vi "niScope Setup Virtual Channels.vi"(4 "samples count":i64=50000 min=1, 6 "fs [Hz]":dbl=50000.0, 7 "trigger setup (Immediate)":T1={"coupling"=1, "level [V]"=0.0, "slope"=0, "mode"=enum."Immediate"} {"level [V]" format="%.2f"; "coupling" items=["AC"=0, "DC"=1, "HF Reject"=3, "LF Reject"=4, "AC Plus HF Reject"=1001]}, 8 "error in":errorcluster, 10 "voltage ranges [Vpk] (empty: use global default)":dbl[](array[numeric]), 11 "niScope in":T4={"channel cfg"=[], "sessions"=[], "multi cards"=FALSE, "channels"=0, "type"=enum."n/a", "memory [B/chn]"=0, "ext. clock [Hz]"=0.0, "samples count"=0, "use streaming"=FALSE, "proc setup"={"packet size [smpl]"=0, "current timeout [s]"=0.0, "blk2blk timeout [s]"=0.0, "event time"=timestamp(0 s since 1904-01-01), "temp sampl T [s]"=0.0, "data queue"=refnum, "stop notifier"=refnum, "proc ref"=refnum}, "sample width [B]"=0, "ranges [V]"=[], "trigger setup"={"coupling"=1, "level [V]"=0.0, "slope"=0, "mode"=enum."Immediate"}, "fs [Hz]"=0.0, "bitres [bit]"=0} {"trigger setup"."level [V]" format="%.2f"; "trigger setup"."coupling" items=["AC"=0, "DC"=1, "HF Reject"=3, "LF Reject"=4, "AC Plus HF Reject"=1001]; "channel cfg"."Range [Vpk]" min=0.0; "channel cfg"."Channel" min=0}) -> (0 "error out":errorcluster, 3 "niScope out":T4={"channel cfg"=[], "sessions"=[], "multi cards"=FALSE, "channels"=0, "type"=enum."n/a", "memory [B/chn]"=0, "ext. clock [Hz]"=0.0, "samples count"=0, "use streaming"=FALSE, "proc setup"={"packet size [smpl]"=0, "current timeout [s]"=0.0, "blk2blk timeout [s]"=0.0, "event time"=timestamp(0 s since 1904-01-01), "temp sampl T [s]"=0.0, "data queue"=refnum, "stop notifier"=refnum, "proc ref"=refnum}, "sample width [B]"=0, "ranges [V]"=[], "trigger setup"={"coupling"=1, "level [V]"=0.0, "slope"=0, "mode"=enum."Immediate"}, "fs [Hz]"=0.0, "bitres [bit]"=0} {"trigger setup"."level [V]" format="%.2f"; "trigger setup"."coupling" items=["AC"=0, "DC"=1, "HF Reject"=3, "LF Reject"=4, "AC Plus HF Reject"=1001]; "channel cfg"."Range [Vpk]" min=0.0; "channel cfg"."Channel" min=0})   [LabVIEW 2018, in "niScope Virtual Digitizer.lvlib"]
doc: "Configures all virtual channels of the digitizer. Uses global and channel settings from the input session. If vector of voltage ranges in assigned to the function it will override default channel setting from the session. If it is empty, the defaults in the session will be used. Sampling rate and samples count to capture are set by additional inputs. Trigger can be set to other than immediate mode only for single shot mode (for streaming mode it is not yet supported). The VI prepares the cards for acquiring the data. It also implements synchronization via ni-Tclk in case multiple cards are used together. Call this at least once before doing first acquisition. It is not necessary to call this again when multiple acquisitions are performed repetedely with identical settings."
uses:
  niScope Virtual Digitizer.lvlib
  niScope Session.ctl
  niScope Virtual Channel Config.ctl
  niScope Virtual Channel Mode.ctl
  niScope Virtual Channel Input Z.ctl
  niScope Virtual Channel Coupling.ctl
  niScope Type.ctl
  niScope Digitizing Process Options.ctl
  niScope Data Packet.ctl
  niScope Trigger Setup.ctl
  <instrlib>/niScope/Controls/niScope trigger coupling.ctl
  <instrlib>/niScope/Controls/niScope trigger slope.ctl
  <instrlib>/niScope/Controls/niScope vertical coupling.ctl
  <instrlib>/niScope/Controls/niScope trigger source.ctl
  <vilib>/Utility/error.llb/Error Cluster From Error Code.vi
  <instrlib>/niScope/Configure/Trigger/niScope Configure Trigger Edge.vi
  <instrlib>/niScope/Configure/Trigger/niScope Configure Trigger Immediate.vi
  <instrlib>/niScope/Configure/Trigger/niScope Configure Trigger Software.vi
  <vilib>/ErrorRing/Error Ring.xnode
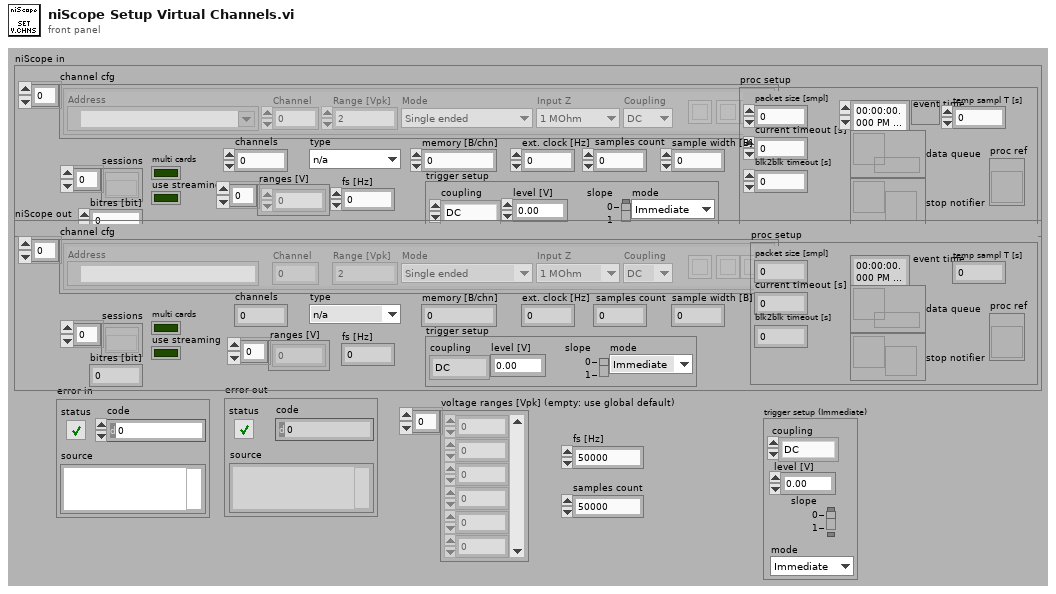
[diagram p1: front panel]
types:
  T1 = typedef "niScope Virtual Digitizer.lvlib/niScope Trigger Setup.ctl" = cluster{"coupling":T2, "level [V]":dbl, "slope":T3, "mode":enum16{"Immediate", "External", "Level"}}
  T2 = typedef "niScope trigger coupling.ctl" = u16
  T3 = typedef "niScope trigger slope.ctl" = i32
  T4 = typedef "niScope Virtual Digitizer.lvlib/niScope Session.ctl" = cluster{"channel cfg":T5[], "sessions":refnum<k20>[], "multi cards":bool, "channels":i32, "type":T9, "memory [B/chn]":i32, "ext. clock [Hz]":dbl, "samples count":i64, "use streaming":bool, "proc setup":T10, "sample width [B]":i32, "ranges [V]":dbl[], "trigger setup":T1, "fs [Hz]":dbl, "bitres [bit]":i32}
  T5 = typedef "niScope Virtual Digitizer.lvlib/niScope Virtual Channel Config.ctl" = cluster{"Address":refnum<k15>, "Channel":i32, "Mode":T6, "Input Z":T7, "Coupling":T8, "Range [Vpk]":dbl, "btn clr":bool, "btn up":bool, "btn down":bool}
  T6 = typedef "niScope Virtual Digitizer.lvlib/niScope Virtual Channel Mode.ctl" = enum16{"Single ended", "Unbal. differential", "Differential"}
  T7 = typedef "niScope Virtual Digitizer.lvlib/niScope Virtual Channel Input Z.ctl" = enum16{"1 MOhm", "50 Ohm"}
  T8 = typedef "niScope Virtual Digitizer.lvlib/niScope Virtual Channel Coupling.ctl" = enum16{"AC", "DC", "GND"}
  T9 = typedef "niScope Virtual Digitizer.lvlib/niScope Type.ctl" = enum16{"n/a", "5922"}
  T10 = typedef "niScope Virtual Digitizer.lvlib/niScope Digitizing Process Options.ctl" = cluster{"packet size [smpl]":i64, "current timeout [s]":dbl, "blk2blk timeout [s]":dbl, "event time":timestamp, "temp sampl T [s]":dbl, "data queue":refnum<queue>, "stop notifier":refnum<notifier>, "proc ref":refnum<vi>}
  T11 = typedef "niScope Virtual Digitizer.lvlib/niScope Physical Cards.ctl" = cluster{"chn lst":i32[], "addr":refnum<k15>, "chn pos":i32[]}
  T12 = typedef "niScope trigger source.ctl" = string
  T13 = typedef "niScope vertical coupling.ctl" = i32
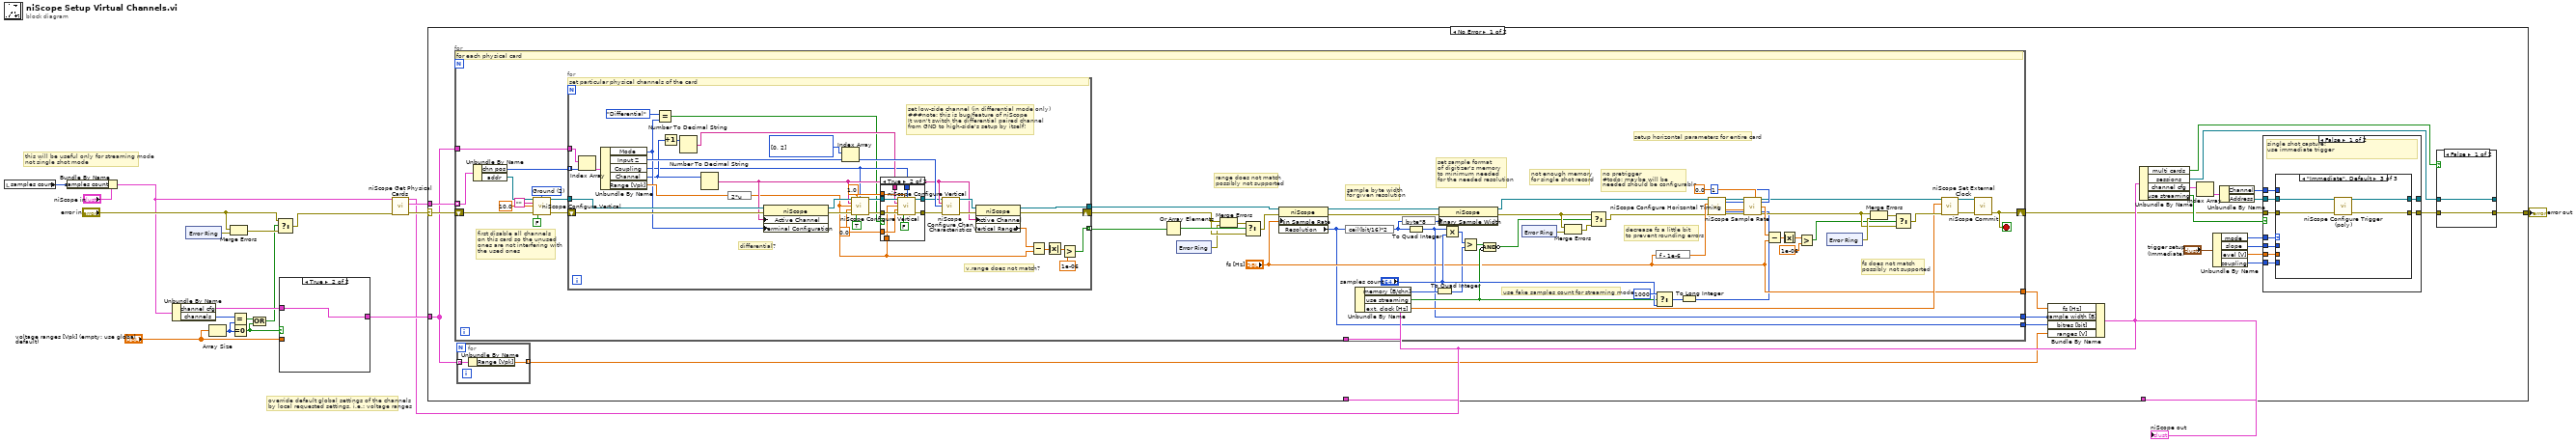
[diagram p0: block diagram]
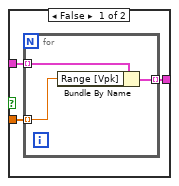
[diagram p2: hidden frame]
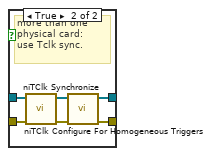
[diagram p3: hidden frame]
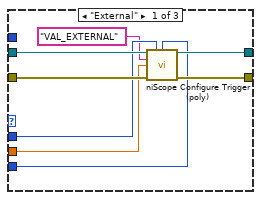
[diagram p4: hidden frame]
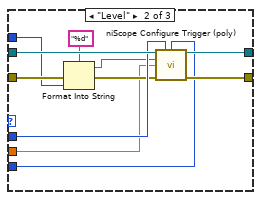
[diagram p5: hidden frame]
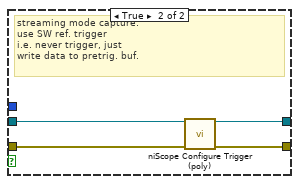
[diagram p6: hidden frame]
diagram:
  # "this will be useful only for streaming mode\nnot single shot mode"
  # "override default global settings of the channels\nby local requested settings, i.e.: voltage ranges"
  n1 = local read "samples count"() -> (w11:i64)
  n2 = Bundle By Name(cluster="niScope in", "samples count"=w11) -> (w9:T4)
  n3 = Unbundle By Name(w9) -> ("channel cfg"=w18:T5[], "channels"=w19:i32)
  n4 = xnode "Error Ring"() -> ("error out"=w15:errorcluster)
  n5 = Array Size(array="voltage ranges [Vpk] (empty: use global default)") -> (size(s)=w6:i32)
  n6 = Merge Errors("error in", w15) -> (w14:errorcluster)
  n7 = Equal?(x=w19, y=w6) -> (x = y?=w7:bool)
  n8 = Equal To 0?(x=w6) -> (x = 0?=w3:bool)
  n9 = Compound Arithmetic op=OR(w7, w3) -> (w5:bool)
  n10 = Select(t="error in", s=w5, f=w14) -> (s? t:f=w2:errorcluster)
  n11 = case shown="True" w3 {
    tunnel: w18 -> [w23 w27]
    tunnel: [w22 w27] -> w17
    tunnel: "voltage ranges [Vpk] (empty: use global default)" -> [w21 _]
    frame False {
      n12 = for {
        tunnel: w23 -> [w26] mode=indexing
        tunnel: w21 -> [w24] mode=indexing
        tunnel: [w25] -> w22 mode=indexing
        n13 = Bundle By Name(cluster=w26, "Range [Vpk]"=w24) -> (w25:T5)
      }
    }
    frame True {
    }
  }
  n14 = call "niScope Get Physical Cards.vi"("error in"=w2, "niScope in"=w9) -> ("error out"=w13:errorcluster, "card list"=w20:T11[], "niScope out"=w8:T4)  [unwired: 7 in]
  n15 = case shown="No Error" w13 {
    selector: w13 -> [w51 w222]
    tunnel: w20 -> [w33 _]
    tunnel: w17 -> [w32 _]
    tunnel: w8 -> [w36 w221]
    tunnel: [w43 w222] -> w10
    tunnel: [w35 w221] -> w1
    frame No Error {
      n16 = for {
        tunnel: w33 -> [w157] mode=indexing
        shift-right: [w128] -> w28
        shift-left: w51 -> [w154]
        tunnel: w32 -> [w148]
        tunnel: w36 -> [w138]
        tunnel: [w102] -> w34
        tunnel: ["fs [Hz]"] -> w30
        tunnel: [w99] -> w29
        stop <- w128 stop-if-true
        w150 = T13 2 items=["AC", "DC", "Ground"] ("vertical coupling")
        # "set sample format\nof digitizer's memory\nto minimum needed\nfor the needed resolution"
        # "not enough memory\nfor single shot record"
        # "sample byte width\nfor given resolution"
        # "use fake samples count for streaming mode"
        # "fs does not match\npossibly not supported"
        # "setup horizontal parameters for entire card"
        # "range does not match\npossibly not supported"
        # "decrease fs a little bit\nto prevent rounding errors"
        # "no pretrigger\n#todo: maybe will be\nneeded should be configurable"
        # "first disable all channels\non this card so the unused\nones are not interfering with\nthe used ones"
        # "for each physical card"
        n17 = Unbundle By Name(w157) -> ("chn pos"=w156:i32[], "addr"=w153:refnum<k15>)
        n18 = call <instrlib>:"niScope Configure Vertical.vi"("instrument handle"=w153, "vertical coupling"=w150, "channels"="", "vertical range"=10.0, "error in"=w154, "channel enabled"=FALSE) -> ("instrument handle out"=w152:refnum<k15>, "error out"=w155:errorcluster)  [unwired: 8 in]
        n19 = for {
          shift-right: [w193] -> w134
          shift-left: w155 -> [w202]
          tunnel: w156 -> [w208] mode=indexing
          tunnel: w152 -> [w201]
          tunnel: w148 -> [w204]
          tunnel: [w192] -> w119
          tunnel: [w191] -> w137 mode=indexing
          w189 = u32[] [0, 2] items=["1 mega ohm"=0, "50 ohms"=2]
          w175 = 0.0 ("vertical offset")
          w177 = 1.0 ("probe attenuation")
          # "set low-side channel (in differential mode only)\n###note: this is bug/feature of niScope\nIt won't switch the differential paired channel\nfrom GND to high-side's setup by itself!"
          # "v.range does not match?"
          # "differential?"
          # "set particular physical channels of the card"
          n20 = Index Array(array=w204, index=w208) -> (element=w207:T5)
          n21 = Unbundle By Name(w207) -> ("Mode"=w187:T6, "Input Z"=w190:T7, "Coupling"=w176:T8, "Channel"=w185:i32, "Range [Vpk]"=w206:dbl)
          n22 = Equal?(x=niScope_Virtual_Channel_Mode."Differential", y=w187) -> (x = y?=w173:bool)
          n23 = Increment(x=w185) -> (x+1=w183:i32)
          n24 = Number To Decimal String(number=w183) -> (decimal integer string=w178:string)  [unwired: 1 in]
          n25 = Number To Decimal String(number=w185) -> (decimal integer string=w184:string)  [unwired: 1 in]
          n26 = expression code="2*u"(w206) -> (w174:dbl)
          n27 = property class="niScope"(reference=w201, error in=w202, "Active Channel"=w184, "Terminal Configuration"=w187) -> (reference out=w200:refnum<k15>, error out=w203:errorcluster)
          n28 = Index Array(array=w189, index=w190) -> (element=w188:u32)
          n29 = call <instrlib>:"niScope Configure Vertical.vi"("instrument handle"=w200, "probe attenuation"=w177, "vertical coupling"=w176, "channels"=w184, "vertical range"=w174, "vertical offset"=w175, "error in"=w203, "channel enabled"=TRUE) -> ("instrument handle out"=w181:refnum<k15>, "error out"=w182:errorcluster)  [unwired: 6 in]
          n30 = case shown="True" w173 {
            tunnel: w182 -> [w209 w220]
            tunnel: w181 -> [w210 w219]
            tunnel: [w209 w218] -> w180
            tunnel: [w210 w217] -> w179
            tunnel: w178 -> [_ w216]
            tunnel: w177 -> [_ w215]
            tunnel: w176 -> [_ w214]
            tunnel: w175 -> [_ w212]
            tunnel: w174 -> [_ w211]
            frame False {
            }
            frame True {
              n31 = call <instrlib>:"niScope Configure Vertical.vi"("instrument handle"=w219, "probe attenuation"=w215, "vertical coupling"=w214, "channels"=w216, "vertical range"=w211, "vertical offset"=w212, "error in"=w220, "channel enabled"=FALSE) -> ("instrument handle out"=w217:refnum<k15>, "error out"=w218:errorcluster)  [unwired: 6 in]
            }
          }
          n32 = call <instrlib>:"niScope Configure Chan Characteristics.vi"("instrument handle"=w179, "channels"=w184, "input impedance"=w188, "error in"=w180) -> ("instrument handle out"=w198:refnum<k15>, "error out"=w199:errorcluster)  [unwired: 10 in]
          n33 = property class="niScope"(reference=w198, error in=w199, "Active Channel"=w184) -> (reference out=w192:refnum<k15>, error out=w193:errorcluster, "Vertical Range"=w197:dbl)
          n34 = Subtract(x=w197, y=w174) -> (x-y=w196:dbl)
          n35 = Absolute Value(x=w196) -> (abs(x)=w195:dbl)
          n36 = Greater?(x=w195, y=1e-06) -> (0:w191:bool)
        }
        n37 = Or Array Elements(Boolean array=w137) -> (logical OR=w136:bool)
        n38 = xnode "Error Ring"() -> ("error out"=w133:errorcluster)
        n39 = Merge Errors(w134, w133) -> (w135:errorcluster)
        n40 = Select(t=w135, s=w136, f=w134) -> (s? t:f=w120:errorcluster)
        n41 = property class="niScope"(reference=w119, error in=w120, "Min Sample Rate"="fs [Hz]") -> (reference out=w109:refnum<k15>, error out=w110:errorcluster, "Resolution"=w99:i32)
        n42 = expression code="ceil(bit/16)*2"(w99) -> (w104:i32)
        n43 = Unbundle By Name(w138) -> ("memory [B/chn]"=w114:i32, "use streaming"=w112:bool, "ext. clock [Hz]"=w124:dbl)
        n44 = expression code="byte*8"(w104) -> (w108:i32)
        n45 = To Quad Integer(1:w104) -> (0:w102:i64)
        n46 = To Quad Integer(1:w114) -> (0:w101:i64)
        n47 = property class="niScope"(reference=w109, error in=w110, "Binary Sample Width"=w108) -> (reference out=w106:refnum<k15>, error out=w107:errorcluster)
        n48 = Multiply(x=w102, y="samples count") -> (x*y=w115:i64)
        n49 = Greater?(x=w115, y=w101) -> (0:w113:bool)
        n50 = Compound Arithmetic op=AND(w113, invert w112) -> (invert w105:bool)
        n51 = xnode "Error Ring"() -> ("error out"=w117:errorcluster)
        n52 = Merge Errors(w107, w117) -> (w118:errorcluster)
        n53 = Select(t=w107, s=w105, f=w118) -> (s? t:f=w111:errorcluster)
        n54 = expression code="f - 1e-6"("fs [Hz]") -> (w143:dbl)
        n55 = Select(t=i64 1000, s=w112, f="samples count") -> (s? t:f=w122:i64)
        n56 = To Long Integer(number=w122) -> (32bit integer=w100:i32)
        n57 = call <instrlib>:"niScope Configure Horizontal Timing.vi"("instrument handle"=w106, "number of records"=1, "min sample rate"=w143, "reference position"=0.0, "error in"=w111, "min record length"=w100) -> ("instrument handle out"=w142:refnum<k15>, "error out"=w141:errorcluster)  [unwired: 8 in]
        n58 = call <instrlib>:"niScope Sample Rate.vi"("instrument handle"=w142, "error in"=w141) -> ("instrument handle out"=w125:refnum<k15>, "actual sample rate"=w144:dbl, "error out"=w130:errorcluster)  [unwired: 11 in]
        n59 = Subtract(x=w144, y="fs [Hz]") -> (x-y=w145:dbl)
        n60 = Absolute Value(x=w145) -> (abs(x)=w146:dbl)
        n61 = Greater?(x=w146, y=1e-06) -> (0:w129:bool)
        n62 = xnode "Error Ring"() -> ("error out"=w132:errorcluster)
        n63 = Merge Errors(w130, w132) -> (w131:errorcluster)
        n64 = Select(t=w131, s=w129, f=w130) -> (s? t:f=w127:errorcluster)
        n65 = call "niScope Set External Clock.vi"("error in"=w127, "ref. clock rate [Hz] (0: use internal clock)"=w124, "niScope reference in"=w125) -> ("error out"=w126:errorcluster, "reference out"=w98:refnum<k15>)  [unwired: 4 in, 3 out]
        n66 = call <instrlib>:"niScope Commit.vi"("instrument handle"=w98, "error in"=w126) -> ("error out"=w128:errorcluster)  [unwired: 12 in, 1 out]
      }
      n67 = for {
        tunnel: w32 -> [w53] mode=indexing
        tunnel: [w52] -> w31 mode=indexing
        n68 = Unbundle By Name(w53) -> ("Range [Vpk]"=w52:dbl)
      }
      n69 = Bundle By Name(cluster=w36, "fs [Hz]"=w30, "sample width [B]"=w34, "bitres [bit]"=w29, "ranges [V]"=w31) -> (w35:T4)
      n70 = Unbundle By Name(w36) -> ("multi cards"=w44:bool, "sessions"=w45:refnum<k20>[], "channel cfg"=w50:T5[], "use streaming"=w47:bool)
      n71 = Index Array(array=w50) -> (element=w49:T5)  [unwired: 1 in]
      n72 = Unbundle By Name("trigger setup (Immediate)") -> ("mode"=w41:enum16{"Immediate", "External", "Level"}, "slope"=w40:T3, "level [V]"=w38:dbl, "coupling"=w37:T2)
      n73 = Unbundle By Name(w49) -> ("Channel"=w39:i32, "Address"=w48:refnum<k15>)
      n74 = case shown="False" w47 {
        tunnel: w28 -> [w70 w97]
        tunnel: w48 -> [w69 w96]
        tunnel: [w68 w95] -> w46
        tunnel: [w67 w94] -> _
        tunnel: w41 -> [w66 _]
        tunnel: w40 -> [w65 _]
        tunnel: w39 -> [w64 _]
        tunnel: w38 -> [w63 _]
        tunnel: w37 -> [w62 _]
        frame False {
          # "single shot capture:\nuse immediate trigger"
          n75 = case shown="\"Immediate\", Default" w66 {
            tunnel: w70 -> [w78 w85 w93]
            tunnel: w69 -> [w77 w89 w92]
            tunnel: [w75 w87 w91] -> w68
            tunnel: [w76 w88 w90] -> w67
            tunnel: w65 -> [w74 w86 _]
            tunnel: w64 -> [_ w81 _]
            tunnel: w63 -> [w72 w80 _]
            tunnel: w62 -> [w71 w79 _]
            frame "External" {
              n76 = call-poly <instrlib>:"niScope Configure Trigger (poly).vi"("instrument handle"=w77, "trigger slope"=w74, "trigger coupling"=w71, "trigger source"=T12 "VAL_EXTERNAL", "trigger level"=w72, "error in"=w78) -> ("instrument handle out"=w76:refnum<k15>, "error out"=w75:errorcluster)  [unwired: 8 in]
            }
            frame "Level" {
              n77 = Format Into String(format string="%d", error in=w85, w81) -> (resulting string=w83:string, error out=w84:errorcluster)  [unwired: 1 in]
              n78 = call-poly <instrlib>:"niScope Configure Trigger (poly).vi"("instrument handle"=w89, "trigger slope"=w86, "trigger coupling"=w79, "trigger source"=w83, "trigger level"=w80, "error in"=w84) -> ("instrument handle out"=w88:refnum<k15>, "error out"=w87:errorcluster)  [unwired: 8 in]
            }
            frame "Immediate", Default {
              n79 = call-poly <instrlib>:"niScope Configure Trigger (poly).vi"("instrument handle"=w92, "error in"=w93) -> ("instrument handle out"=w90:refnum<k15>, "error out"=w91:errorcluster)  [unwired: 12 in]
            }
          }
        }
        frame True {
          # "streaming mode capture:\nuse SW ref. trigger\ni.e. never trigger, just\nwrite data to pretrig. buf."
          n80 = call-poly <instrlib>:"niScope Configure Trigger (poly).vi"("instrument handle"=w96, "error in"=w97) -> ("instrument handle out"=w94:refnum<k15>, "error out"=w95:errorcluster)  [unwired: 12 in]
        }
      }
      n81 = case shown="False" w44 {
        tunnel: [w55 w60] -> w43
        tunnel: w46 -> [w55 w59]
        tunnel: w45 -> [w54 w58]
        tunnel: [w54 w56] -> _
        frame False {
        }
        frame True {
          # "more than one\nphysical card:\nuse Tclk sync."
          n82 = call <instrlib>:"niTClk Configure For Homogeneous Triggers.vi"("error in (no error)"=w59, "sessions"=w58) -> ("error out"=w61:errorcluster, "sessions out"=w57:refnum<k20>[])  [unwired: 8 in]
          n83 = call <instrlib>:"niTClk Synchronize.vi"("error in (no error)"=w61, "sessions"=w57) -> ("error out"=w60:errorcluster, "sessions out"=w56:refnum<k20>[])  [unwired: 8 in]
        }
      }
    }
    frame Error {
    }
  }
  "error out" <- w10
  "niScope out" <- w1
